vi "CANOpen_Get xPDO Data Refs.vi"(7 "xPDOs GUID":string, 8 "error in (no error)":errorcluster, 10 "State Variables":T6 {"Child Refs" format="%.0x"}, 11 "Section Ref in":T5 format="%.0x") -> (0 "error out":errorcluster, 1 "xPDOs":T1[](array[typedef]) {"PDO Channel" items=["PDO 1", "PDO 2", "PDO 3", "PDO 4"]; "Parameters"."Bit Offset" max=8 step=1; "Parameters"."Byte Offset" max=8 step=1}, 2 "xPDOs Out":T6 {"Child Refs" format="%.0x"}, 3 "Section Ref out":T5 format="%.0x")   [LabVIEW 2021, in "CANOpen Addon Engine.lvlib"]
uses:
  CANOpen Addon Engine.lvlib
  <vilib>/NI VeriStand/Custom Device API/Custom Device Item Ref.ctl
  CANOpen_xPDO VS Refs.ctl
  Shared/CANOpen_PDO Settings.ctl
  Shared/CANOpen_PDO Parameter Settings.ctl
  Shared/CANOpen_PDO Data Type.ctl
  Shared/CANopen Byte Order.ctl
  Shared/CANOpen Addon GUID Lookup Global.vi
  <vilib>/NI VeriStand/Custom Device Tools/Custom Device Utility Library/NI VeriStand - Search for Item by GUID.vi
  <vilib>/NI VeriStand/Custom Device Tools/Custom Device Utility Library/NI VeriStand - Search for All Items by GUID.vi
  <vilib>/NI VeriStand/Custom Device API/Get Item Property (Variant).vi
  <vilib>/NI VeriStand/Custom Device API/Custom Device API.lvlib
  <vilib>/NI VeriStand/Custom Device Tools/Custom Device Utility Library/Custom Device Utility Library.lvlib
  Shared/CANOpen Addon Shared.lvlib
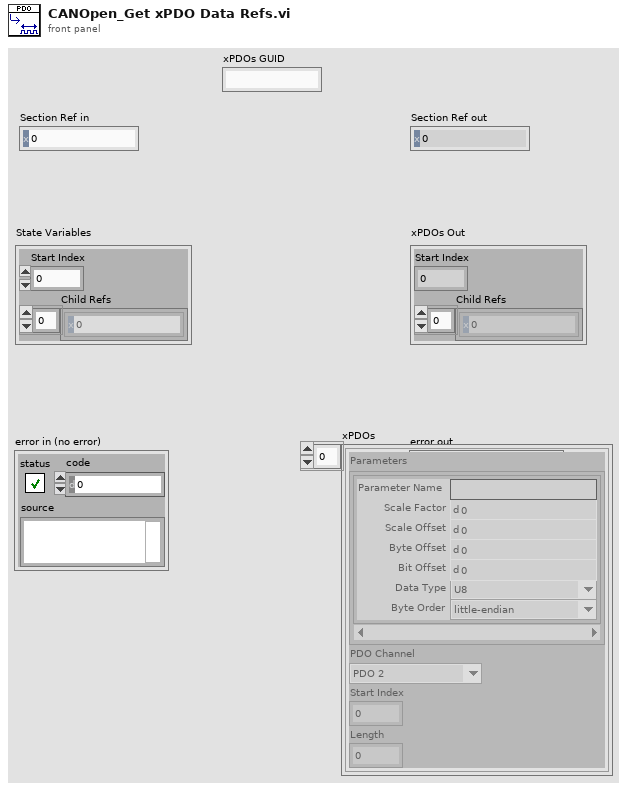
[diagram p1: front panel]
types:
  T1 = typedef "CANOpen Addon Shared.lvlib/CANOpen_PDO Settings.ctl" = cluster{"Parameters":T2[], "PDO Channel":u8, "Start Index":u32, "Length":u32}
  T2 = typedef "CANOpen Addon Shared.lvlib/CANOpen_PDO Parameter Settings.ctl" = cluster{"Parameter Name":string, "Scale Factor":dbl, "Scale Offset":dbl, "Byte Offset":u8, "Bit Offset":u8, "Data Type":T3, "Byte Order":T4}
  T3 = typedef "CANOpen Addon Shared.lvlib/CANOpen_PDO Data Type.ctl" = enum16{"U8", "U16", "U32", "I8", "I16", "I32", "Single", "Double", "Boolean"}
  T4 = typedef "CANOpen Addon Shared.lvlib/CANopen Byte Order.ctl" = enum16{"big-endian network order", "little-endian"}
  T5 = typedef "Custom Device API.lvlib/Custom Device Item Ref.ctl" = u64
  T6 = typedef "CANOpen Addon Engine.lvlib/CANOpen_xPDO VS Refs.ctl" = cluster{"Start Index":i32, "Child Refs":T5[]}
  T7 = typedef "Custom Device API.lvlib/Custom Device Item Info.ctl" = cluster{"Name":string, "Is Channel":bool, "GUID":string, "Is Waveform":bool}
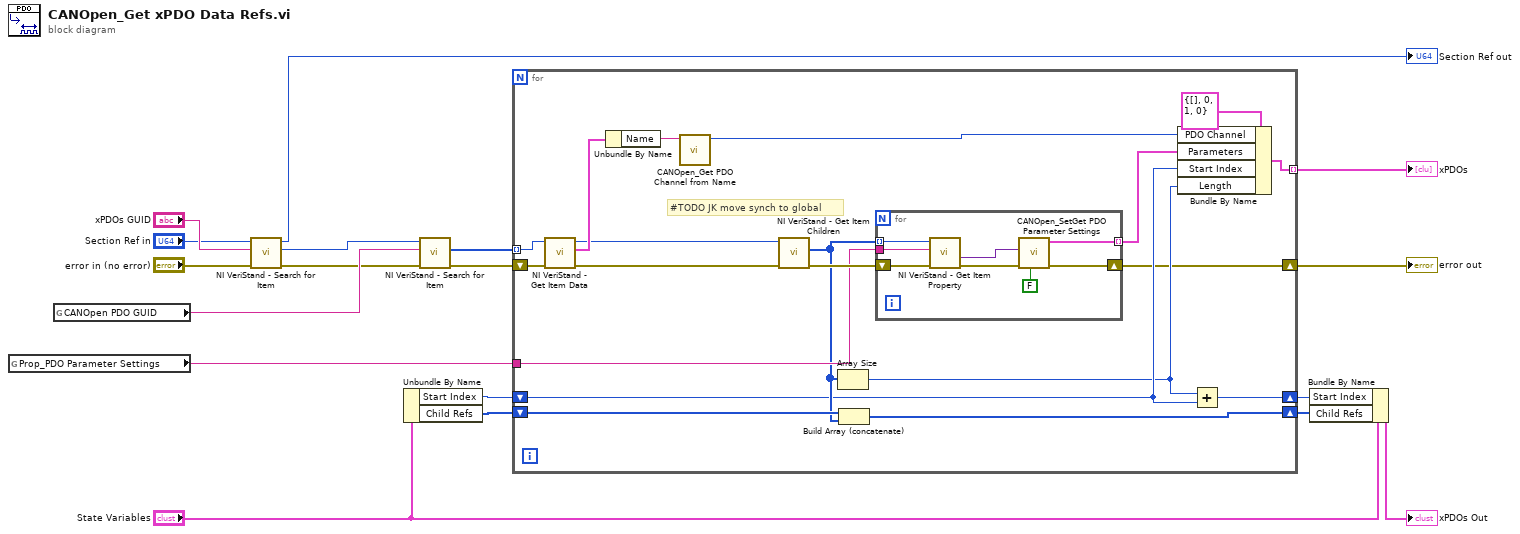
[diagram p0: block diagram]
diagram:
  n1 = global read "CANOpen Addon GUID Lookup Global.vi" "Prop_PDO Parameter Settings"() -> (w4:string)
  n2 = global read "CANOpen Addon GUID Lookup Global.vi" "CANOpen PDO GUID"() -> (w15:string)
  n3 = call-poly <vilib>:"NI VeriStand - Search for Item.vi"("error in"="error in (no error)", "Item GUID"="xPDOs GUID", "Section Ref in"="Section Ref in") -> ("error out"=w14:errorcluster, "Item Ref"=w13:T5, "Section Ref out"=→"Section Ref out":T5)  [unwired: 5 in, 1 out]
  n4 = Unbundle By Name("State Variables") -> ("Start Index"=w11:i32, "Child Refs"=w10:T5[])
  n5 = call-poly <vilib>:"NI VeriStand - Search for Item.vi"("error in"=w14, "Item GUID"=w15, "Section Ref in"=w13) -> ("error out"=w17:errorcluster, "Item Refs"=w16:T5[])  [unwired: 5 in, 2 out]
  n6 = for {
    tunnel: w16 -> [w28] mode=indexing
    shift-right: [w21] -> w12
    shift-left: w17 -> [w27]
    shift-right: [w36] -> w7
    shift-left: w11 -> [w24]
    shift-right: [w35] -> w8
    shift-left: w10 -> [w34]
    tunnel: w4 -> [w31]
    tunnel: [w29] -> w3 mode=indexing
    # "#TODO JK move synch to global"
    n7 = call <vilib>:"NI VeriStand - Get Item Data.vi"("error in (no error)"=w27, "Item Ref in"=w28) -> ("error out"=w19:errorcluster, "Item Info"=w37:T7, "Item Ref out"=w20:T5)  [unwired: 6 in, 1 out]
    n8 = Unbundle By Name(w37) -> ("Name"=w33:string)
    n9 = call "CANOpen_Get PDO Channel from Name.vi"("PDO Channel Name"=w33) -> ("PDO Channel"=w30:i32)  [unwired: 10 in]
    n10 = call <vilib>:"NI VeriStand - Get Item Children.vi"("error in (no error)"=w19, "Item Ref in"=w20) -> ("error out"=w32:errorcluster, "Child Refs"=w26:T5[])  [unwired: 6 in, 2 out]
    n11 = Array Size(array=w26) -> (size(s)=w23:i32)
    n12 = Build Array (concatenate)(w34, w26) -> (w35:T5[])
    n13 = for {
      tunnel: w26 -> [w45] mode=indexing
      shift-right: [w40] -> w21
      shift-left: w32 -> [w44]
      tunnel: w31 -> [w43]
      tunnel: [w38] -> w25 mode=indexing
      n14 = call-poly <vilib>:"NI VeriStand - Get Item Property.vi"("error in (no error)"=w44, "Property Name"=w43, "Item Ref in"=w45) -> ("error out"=w41:errorcluster, "Value"=w39:variant)  [unwired: 5 in, 2 out]
      n15 = call "CANOpen_SetGet PDO Parameter Settings.vi"("Set Parameters"=FALSE, "error in (no error)"=w41, "Parameters"=w39) -> ("error out"=w40:errorcluster, "PDO Parameter Settings out"=w38:T2)  [unwired: 6 in, 1 out]
    }
    n16 = Bundle By Name(cluster=T1 {"Parameters"=[], "PDO Channel"=0, "Start Index"=1, "Length"=0} ("PDO Settings"), "PDO Channel"=w30, "Parameters"=w25, "Start Index"=w24, "Length"=w23) -> (w29:T1)
    n17 = Add(x=w23, y=w24) -> (x+y=w36:i32)
  }
  "error out" <- w12
  "xPDOs" <- w3
  n18 = Bundle By Name(cluster="State Variables", "Start Index"=w7, "Child Refs"=w8) -> (→"xPDOs Out":T6)
